vi "polar-view.vi"() -> ()   [LabVIEW 2017]
uses:
  <vilib>/Math Plots/2D Math Plots/2D Compass/2D Compass Datatype/2D Compass Datatype.lvclass
  <vilib>/Math Plots/2D Math Plots/2D Compass/2D Compass Datatype/Public/Plot Helper (Vector).vi
  <vilib>/Math Plots/2D Math Plots/2D Compass/2D Compass XCtrl/2D Compass.xctl
panel:
  out "Current value":dbl
  in  "stop":bool
  out "2D Compass":refnum<class "2D Plot Datatype.lvclass">[](xcontrol)
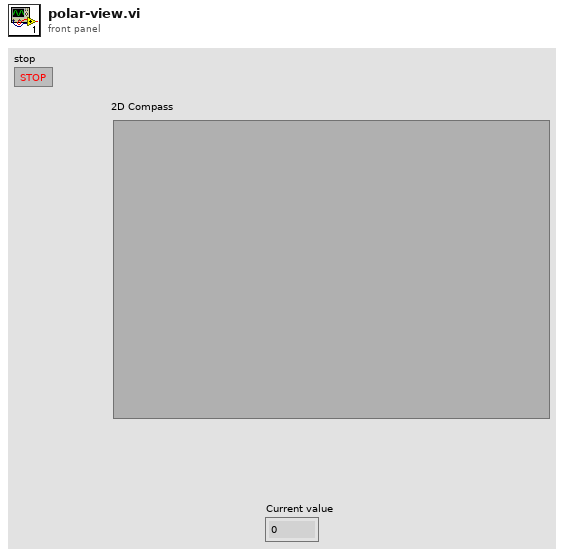
[diagram p1: front panel]
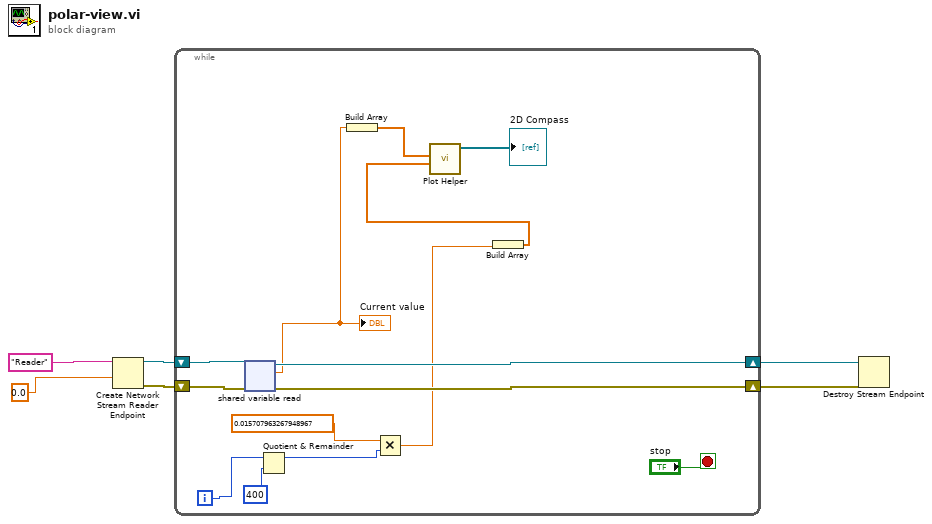
[diagram p0: block diagram]
diagram:
  n1 = Create Network Stream Reader Endpoint(9:0.0, 11:"Reader" ("reader name")) -> (0:w3:errorcluster, 3:w5:refnum<k21>)  [unwired: 5 in]
  n2 = while {
    shift-right: [w17] -> w4
    shift-left: w5 -> [w18]
    shift-right: [w15] -> w2
    shift-left: w3 -> [w16]
    i -> [w12]
    stop <- "stop" stop-if-true
    n3 = shared-variable-read(w18, w16) -> (w17:refnum<k21>, w15:errorcluster, w14:dbl)  [unwired: 1 in, 1 out]
    "Current value" <- w14
    n4 = Quotient & Remainder(x=w12, y=400) -> (x-y*floor(x/y)=w9:i32)  [unwired: 1 out]
    n5 = Build Array(w14) -> (w13:dbl[])
    n6 = Multiply(x=0.015707963267948967, y=w9) -> (x*y=w8:dbl)
    n7 = Build Array(w8) -> (w7:dbl[])
    n8 = call-poly <vilib>:"Plot Helper.vi"("radius vector"=w7, "theta vector"=w13) -> ("2D Plot Class Obj Array out"=→"2D Compass":refnum<class "2D Plot Datatype.lvclass">[])  [unwired: 2 in, 7 out]
  }
  n9 = Destroy Stream Endpoint(8:w2, 11:w4) -> ()  [unwired: 1 out]
